vi "Brake Rack Set.vi"(8 "error in":errorcluster, 9 "Torque":dbl format="%#_13g", 10 "Velocity":dbl format="%#_13g", 11 "queue":refnum<queue>) -> (0 "error out":errorcluster, 3 "dup Message Queue":refnum<queue>)   [LabVIEW 2026, in "Acquisition.lvlib"]
uses:
  Acquisition/Acquisition.lvlib
  support/Message Queue/Message Cluster.ctl
  support/Message Queue/Enqueue Message (Single).vi
  support/Message Queue/Message Queue.lvlib
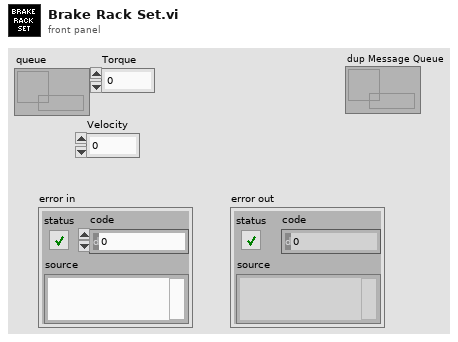
[diagram p1: front panel]
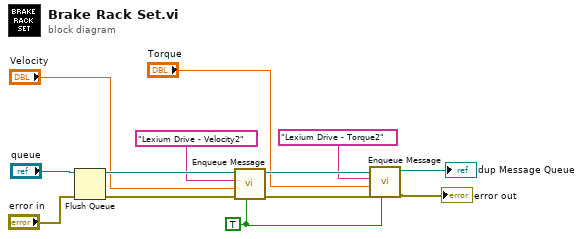
[diagram p0: block diagram]
diagram:
  w3 = TRUE ("Priority Message? (F)")
  n1 = Flush Queue(queue="queue", error in (no error)="error in") -> (queue out=w12:refnum<queue>, error out=w11:errorcluster)  [unwired: 1 out]
  n2 = call-poly "Enqueue Message.vi"("Priority Message? (F)"=w3, "error in (no error)"=w11, "Message Data"="Velocity", "Message"="Lexium Drive - Velocity2", "Message Queue"=w12) -> ("error out"=w8:errorcluster, "dup Message Queue"=w7:refnum<queue>)  [unwired: 5 in]
  n3 = call-poly "Enqueue Message.vi"("Priority Message? (F)"=w3, "error in (no error)"=w8, "Message Data"="Torque", "Message"="Lexium Drive - Torque2", "Message Queue"=w7) -> ("error out"=→"error out":errorcluster, "dup Message Queue"=→"dup Message Queue":refnum<queue>)  [unwired: 5 in]
